vi "fix5035ErrorBug.vi"(8 "error in (no error)":errorcluster, 11 "AndorIKonTempController in":refnum<class "AndorIKonTempController.lvclass">) -> (0 "error out":errorcluster, 3 "AndorIKonTempController out":refnum<class "AndorIKonTempController.lvclass">)   [LabVIEW 2011, in "Hardware.lvlib" / "Channels.lvlib" / "AndorIKonTempController.lvclass"]
uses:
  AndorIKonTempController.lvclass
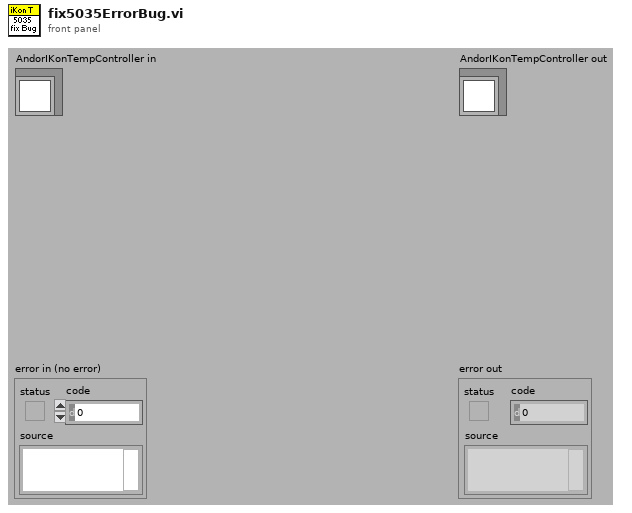
[diagram p1: front panel]
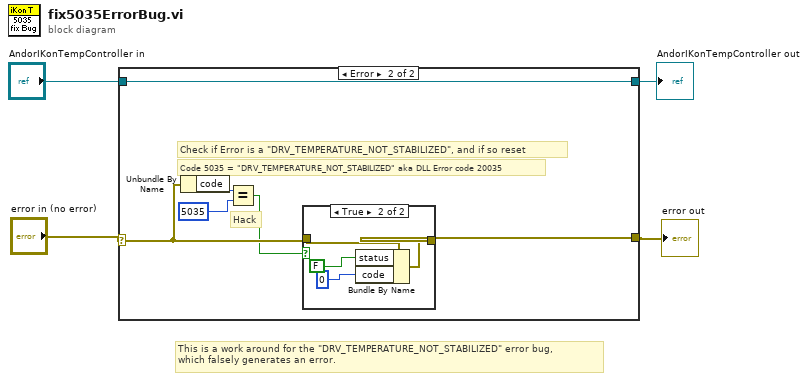
[diagram p0: block diagram]
diagram:
  # "This is a work around for the \"DRV_TEMPERATURE_NOT_STABILIZED\" error bug, \nwhich falsely generates an error."
  n1 = case shown="Error" "error in (no error)" {
    selector: "error in (no error)" -> [w6 w12]
    tunnel: [w6 w8] -> w3
    tunnel: "AndorIKonTempController in" -> [w5 w7]
    tunnel: [w5 w7] -> w1
    frame No Error {
      # "If no error is generated do nothing."
    }
    frame Error {
      # "Code 5035 = \"DRV_TEMPERATURE_NOT_STABILIZED\" aka DLL Error code 20035"
      # "Check if Error is a \"DRV_TEMPERATURE_NOT_STABILIZED\", and if so reset"
      # "Hack"
      n2 = Unbundle By Name(w12) -> ("code"=w10:i32)
      n3 = Equal?(x=w10, y=5035) -> (x = y?=w9:bool)
      n4 = case shown="True" w9 {
        tunnel: w12 -> [w13 w17]
        tunnel: [w13 w14] -> w8
        frame False {
        }
        frame True {
          n5 = Bundle By Name(cluster=w17, "status"=FALSE, "code"=0) -> (w14:errorcluster)
        }
      }
    }
  }
  "error out" <- w3
  "AndorIKonTempController out" <- w1
